vi "七段顯示器分享.vi"() -> ()   [LabVIEW 2014]
uses:
  Main Enum.ctl
  <vilib>/Utility/miscctls.llb/LVMinMaxIncTypeDef.ctl
panel:
  in  "stop":bool
  out "七段顯示器":T1
  in  "Input Number":i32 min=0 max=9
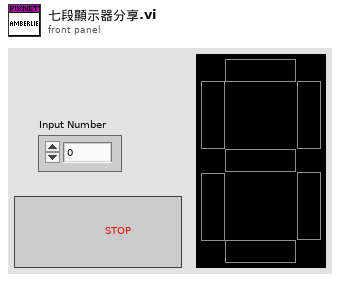
[diagram p1: front panel]
types:
  T1 = cluster{"Boolean":bool, "Boolean 2":bool, "Boolean 3":bool, "Boolean 4":bool, "Boolean 6":bool, "Boolean 7":bool, "Boolean 5":bool}
  T2 = typedef "Main Enum.ctl" = enum16{"Initialize", "Idle", "選擇"}
  T3 = typedef "LVMinMaxIncTypeDef.ctl" = cluster{"Minimum":dbl, "Maximum":dbl, "Increment":dbl}
  T4 = cluster{"Boolean array[0]":bool, "Boolean array[1]":bool, "Boolean array[2]":bool, "Boolean array[3]":bool, "Boolean array[4]":bool, "Boolean array[5]":bool, "Boolean array[6]":bool}
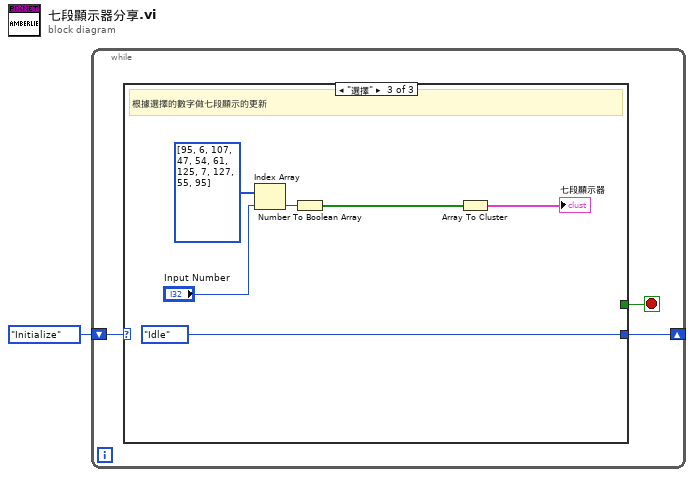
[diagram p0: block diagram]
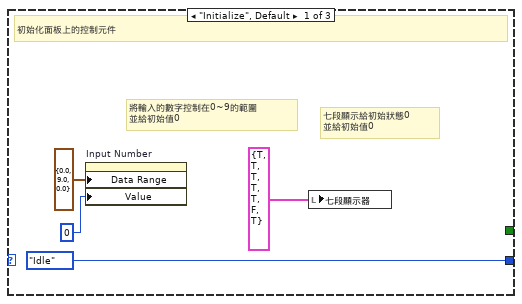
[diagram p2: hidden frame]
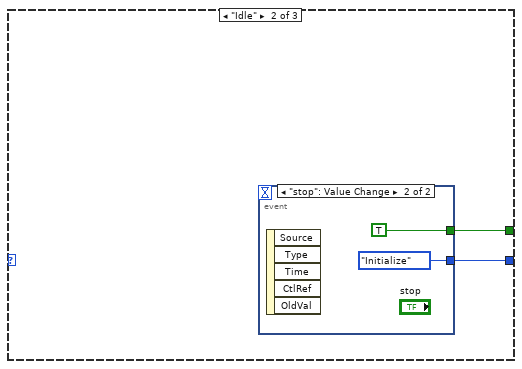
[diagram p3: hidden frame]
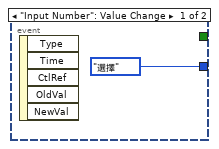
[diagram p4: hidden frame]
diagram:
  n1 = while {
    shift-right: [w4] -> _
    shift-left: Main_Enum."Initialize" -> [w3]
    stop <- w2 stop-if-true
    n2 = case shown="\"選擇\"" w3 {
      tunnel: [Main_Enum."Idle" w10 Main_Enum."Idle"] -> w4
      tunnel: [_ w9 _] -> w2
      frame "Initialize", Default {
        # "七段顯示給初始狀態0\n並給初始值0"
        # "將輸入的數字控制在0~9的範圍\n並給初始值0"
        # "初始化面板上的控制元件"
        n3 = property on="Input Number" class="DigNum (strict)"("Data Range"=T3 {"Minimum"=0.0, "Maximum"=9.0, "Increment"=0.0} ("Data Entry Limits"), "Value"=0 ("Input Number")) -> ()  [unwired: 2 in, 2 out]
        n4 = local write "七段顯示器"(T1 {"Boolean"=TRUE, "Boolean 2"=TRUE, "Boolean 3"=TRUE, "Boolean 4"=TRUE, "Boolean 6"=TRUE, "Boolean 7"=FALSE, "Boolean 5"=TRUE} ("Indicator")) -> ()
      }
      frame "Idle" {
        n5 = event shown="[1] \"stop\": Value Change" {
          selector: _ -> [_ _]
          dyn-events: _ -> [_ _]
          timeout: _ -> [_ _]
          tunnel: [Main_Enum."選擇" Main_Enum."Initialize"] -> w10
          tunnel: [_ TRUE] -> w9
          event "Input Number": Value Change {
            n6 = event-data() -> ()  [unwired: 1 in, 5 out]
          }
          event "stop": Value Change {
            n7 = event-data() -> ()  [unwired: 1 in, 5 out]
          }
        }
      }
      frame "選擇" {
        # "根據選擇的數字做七段顯示的更新"
        n8 = Index Array(array=i32[] [95, 6, 107, 47, 54, 61, 125, 7, 127, 55, 95], index="Input Number") -> (element=w14:i32)
        n9 = Number To Boolean Array(number=w14) -> (Boolean array=w19:bool[])
        n10 = Array To Cluster(array=w19) -> (cluster=→"七段顯示器":T4)
      }
    }
  }
